vi "Check for LabVIEW File.vi"(8 "error in":errorcluster, 10 "File Index":i32, 11 "Peer Review in":refnum<class "Peer Review.lvclass">) -> (0 "error out":errorcluster, 3 "Peer Review out":refnum<class "Peer Review.lvclass">)   [LabVIEW 2020, in "Peer Review.lvclass"]
uses:
  Peer Review.lvclass
  Peer Review.lvclass/Peer Review.ctl
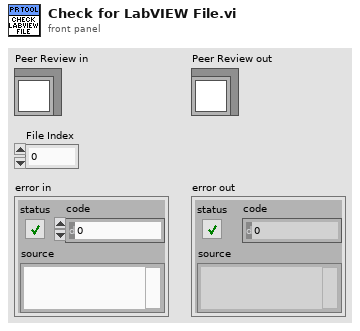
[diagram p1: front panel]
types:
  T1 = typedef "Peer Review.lvclass/File Info.ctl" = cluster{"File ID":i32, "Commit ID":i32, "Reviewed Hash":string, "Relative Path":string, "File Path":path, "File Checksum":string, "State":T2, "FP Changes":i32, "BD Changes":i32, "FP Bounds Error":dbl, "BD Bounds Error":dbl, "Lines Added":i32, "Lines Removed":i32, "Analysis Passes":i32, "Analysis Fails":i32, "Attribute Changes":i32, "Reentrancy State":string, "Cyclomatic Complexity":i32, "Node Count":i32, "Revision Number":u32, "LabVIEW Version":string, "Description":string, "Master Path":path, "Master Checksum":string, "VI Type":T3, "LabVIEW File":bool, "Review Complete":bool, "File Ref":refnum<vi>, "Master Revision":u32}
  T2 = typedef "Peer Review.lvclass/File State.ctl" = enum16{"Interrogation Needed", "Modified", "Deleted", "Added", "Matches Previous", "No Changes", "Moved", "Empty File"}
  T3 = typedef "Peer Review.lvclass/VI Type.ctl" = enum32{"invalid VI type", "Standard VI", "Control VI", "Global VI", "Polymorphic VI", "Configuration VI", "SubSystem", "Facade VI", "Method VI", "Statechart Diagram VI"}
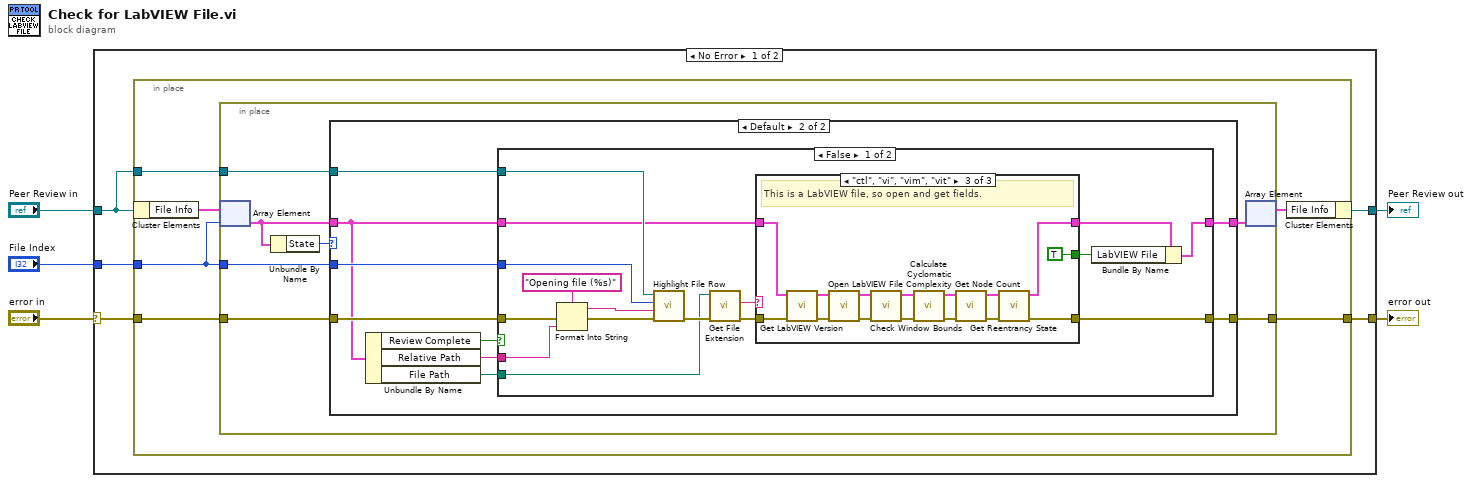
[diagram p0: block diagram]
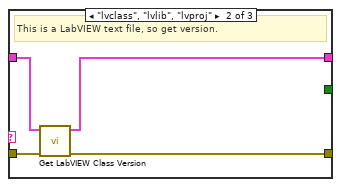
[diagram p4: hidden frame]
diagram:
  n1 = case shown="No Error" "error in" {
    selector: "error in" -> [w9 w75]
    tunnel: [w10 w75] -> w4
    tunnel: "Peer Review in" -> [w7 w74]
    tunnel: [w6 w74] -> w2
    tunnel: "File Index" -> [w8 _]
    frame No Error {
      n2 = in-place "In Place Element Structure" {
        in-place-border: [w16] -> w10
        in-place-border: w9 -> [w15]
        in-place-border: w7 -> [w14]
        in-place-border: w8 -> [w12]
        n3 = in-place-cluster #1(w7) -> ("File Info"=w13:T1[])
        n4 = in-place "In Place Element Structure" {
          in-place-border: [w23] -> w16
          in-place-border: w15 -> [w22]
          in-place-border: w14 -> [w21]
          in-place-border: w12 -> [w20]
          n5 = in-place-array #2(w13, w12) -> (w18:T1)
          n6 = Unbundle By Name(w18) -> ("State"=w19:T2)
          n7 = case shown="Default" w19 {
            tunnel: [w25 w34] -> w23
            tunnel: w22 -> [w25 w33]
            tunnel: w21 -> [_ w32]
            tunnel: w18 -> [w24 w27]
            tunnel: w20 -> [_ w29]
            tunnel: [w24 w28] -> w17
            frame "Deleted" {
            }
            frame Default {
              n8 = Unbundle By Name(w27) -> ("Review Complete"=w26:bool, "Relative Path"=w31:string, "File Path"=w30:path)
              n9 = case shown="False" w26 {
                tunnel: [w50 w73] -> w34
                tunnel: w33 -> [w49 w73]
                tunnel: w32 -> [w48 _]
                tunnel: w31 -> [w42 _]
                tunnel: w30 -> [w41 _]
                tunnel: w29 -> [w40 _]
                tunnel: [w36 w72] -> w28
                tunnel: w27 -> [w39 w72]
                frame False {
                  n10 = Format Into String(format string="Opening file (%s)", error in=w49, w42) -> (resulting string=w45:string, error out=w46:errorcluster)  [unwired: 1 in]
                  n11 = call "Highlight File Row.vi"("error in"=w46, "Status"=w45, "Current Row"=w40, "Peer Review"=w48) -> ("error out"=w43:errorcluster)  [unwired: 7 in]
                  n12 = call <vilib>:"Get File Extension.vi"("error in (no error)"=w43, "file"=w41) -> ("error out"=w47:errorcluster, "lowercase file extension"=w38:string)  [unwired: 5 in, 3 out]
                  n13 = case shown="\"ctl\", \"vi\", \"vim\", \"vit\"" w38 {
                    tunnel: [w52 w56 w57] -> w50
                    tunnel: w47 -> [w52 w55 w62]
                    tunnel: w39 -> [w51 w53 w64]
                    tunnel: [w51 w54 w59] -> w37
                    tunnel: [_ _ TRUE] -> w35
                    frame Default {
                      # "This is not a LabVIEW file, so do nothing."
                    }
                    frame "lvclass", "lvlib", "lvproj" {
                      # "This is a LabVIEW text file, so get version."
                      n14 = call "Get LabVIEW Class Version.vi"("error in"=w55, "File Info in"=w53) -> ("error out"=w56:errorcluster, "File Info out"=w54:T1)  [unwired: 8 in]
                    }
                    frame "ctl", "vi", "vim", "vit" {
                      # "This is a LabVIEW file, so open and get fields."
                      n15 = call "Get LabVIEW Version.vi"("error in"=w62, "File Info in"=w64) -> ("error out"=w63:errorcluster, "File Info out"=w65:T1)  [unwired: 8 in]
                      n16 = call "Open LabVIEW File.vi"("error in"=w63, "File Info in"=w65) -> ("error out"=w71:errorcluster, "File Info out"=w69:T1)  [unwired: 8 in]
                      n17 = call "Check Window Bounds.vi"("error in"=w71, "File Info in"=w69) -> ("error out"=w70:errorcluster, "File Info out"=w68:T1)  [unwired: 8 in]
                      n18 = call "Calculate Cyclomatic Complexity.vi"("error in"=w70, "File Info in"=w68) -> ("error out"=w67:errorcluster, "File Info out"=w66:T1)  [unwired: 8 in]
                      n19 = call "Get Node Count.vi"("error in"=w67, "File Info in"=w66) -> ("error out"=w58:errorcluster, "File Info out"=w60:T1)  [unwired: 8 in]
                      n20 = call "Get Reentrancy State.vi"("error in"=w58, "File Info in"=w60) -> ("error out"=w57:errorcluster, "File Info out"=w59:T1)  [unwired: 8 in]
                    }
                  }
                  n21 = Bundle By Name(cluster=w37, "LabVIEW File"=w35) -> (w36:T1)
                }
                frame True {
                  # "File has already been reviewed, so do nothing."
                }
              }
            }
          }
          n22 = in-place-array #2(w17) -> (w11:T1[])  [unwired: 1 out]
        }
        n23 = in-place-cluster #1("File Info"=w11) -> (w6:refnum<class "Peer Review.lvclass">)
      }
    }
    frame Error {
    }
  }
  "Peer Review out" <- w2
  "error out" <- w4
